vi "Alarma_EN50160_G02.vi"() -> ()   [LabVIEW 2018]
uses:
  Global/PQ_flags.vi
  Global/Alarmas_indicadores-LED.vi
  Global/estadoGeneradores.vi
  Global/Demo.vi
panel:
  in  "type specifier VI Refnum (for type only) 5":refnum<vi>
  in  "type specifier VI Refnum (for type only) 4":refnum<vi>
  in  "type specifier VI Refnum (for type only) 3":refnum<vi>
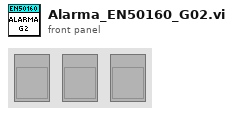
[diagram p1: front panel]
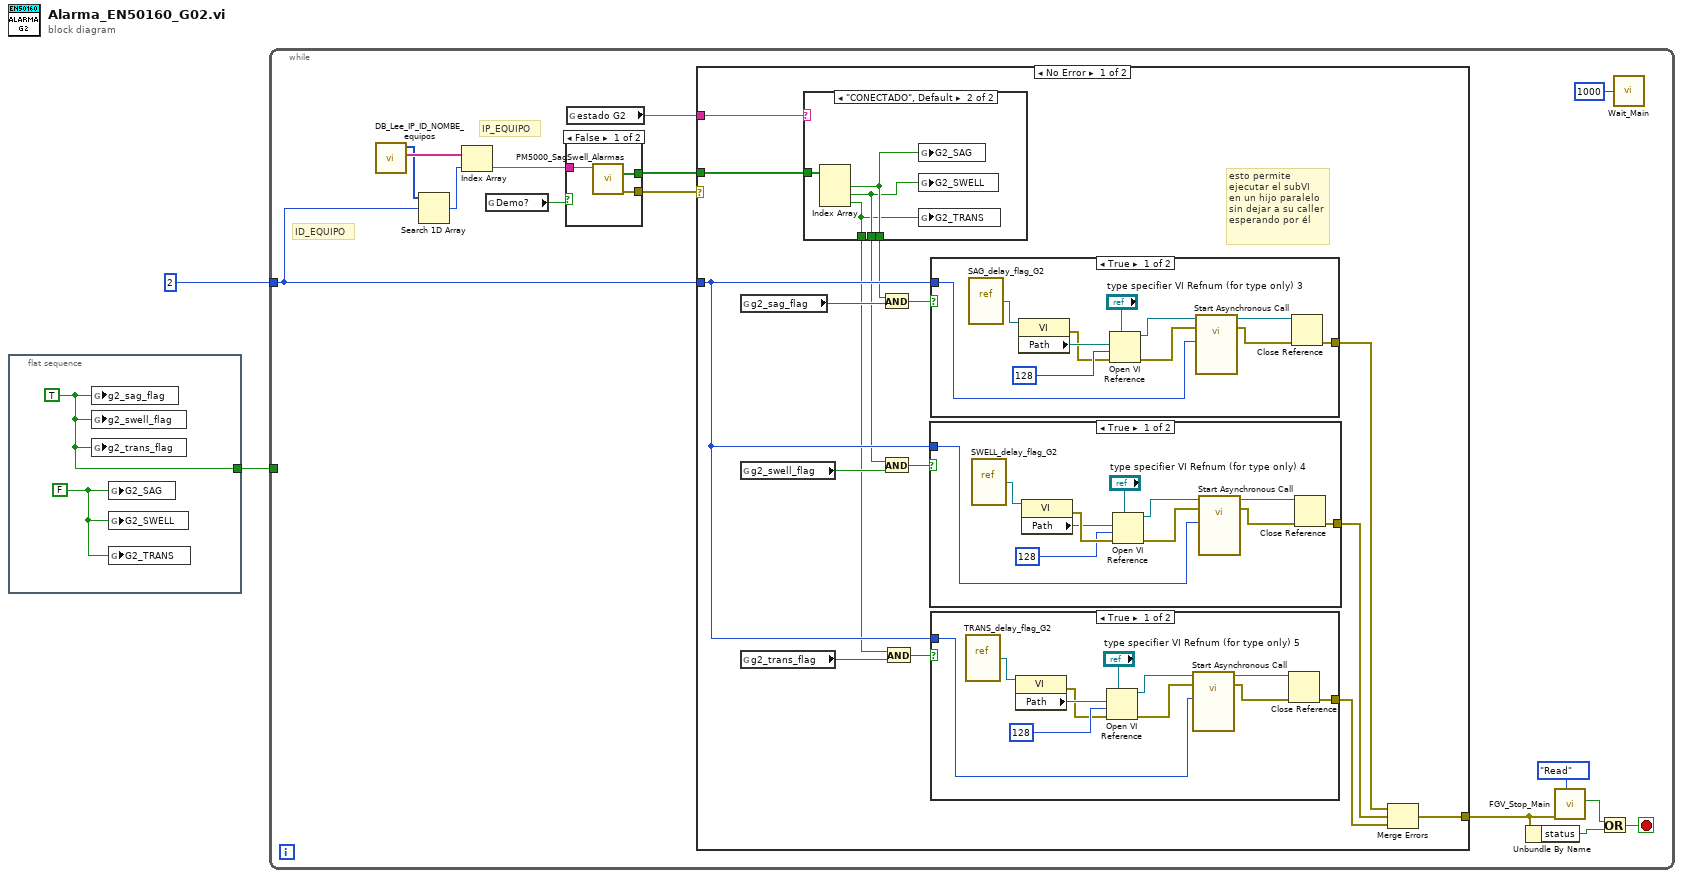
[diagram p0: block diagram]
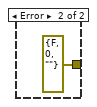
[diagram p6: hidden frame]
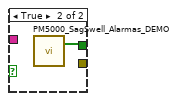
[diagram p7: hidden frame]
diagram:
  n1 = flat-sequence {
    tunnel: [w4] -> w2
    frame #0 {
      w3 = FALSE ("G1_SAG")
      w4 = TRUE ("sag_flag")
      n2 = global write "PQ_flags.vi" "g2_sag_flag"(w4) -> ()
      n3 = global write "PQ_flags.vi" "g2_swell_flag"(w4) -> ()
      n4 = global write "PQ_flags.vi" "g2_trans_flag"(w4) -> ()
      n5 = global write "Alarmas_indicadores-LED.vi" "G2_SAG"(w3) -> ()
      n6 = global write "Alarmas_indicadores-LED.vi" "G2_SWELL"(w3) -> ()
      n7 = global write "Alarmas_indicadores-LED.vi" "G2_TRANS"(w3) -> ()
    }
  }
  n8 = while {
    tunnel: w2 -> [_]
    tunnel: 2 ("element") -> [w6]
    stop <- w11 stop-if-true
    # "IP_EQUIPO"
    # "ID_EQUIPO"
    n9 = call "DB_Lee_IP_ID_NOMBE_equipos.vi"() -> ("IP_EQUIPO"=w18:string[], "ID_EQUIPO"=w16:i32[])  [unwired: 8 in, 2 out]
    n10 = Search 1D Array(1D array=w16, element=w6) -> (index of element=w17:i32)  [unwired: 1 in]
    n11 = Index Array(array=w18, index=w17) -> (element=w15:string)
    n12 = global read "Demo.vi" "Demo?"() -> (w5:bool)
    n13 = case shown="False" w5 {
      tunnel: [w76 w77] -> w19
      tunnel: w15 -> [w75 _]
      tunnel: [w74 _] -> w7
      frame False {
        n14 = call "PM5000_SagSwell_Alarmas.vi"("Network Path"=w75) -> ("error out"=w74:errorcluster, "PQ_Alarmas"=w76:bool[])  [unwired: 8 in, 1 out]
      }
      frame True {
        n15 = call "PM5000_SagSwell_Alarmas_DEMO.vi"() -> ("PQ_Alarmas 2"=w77:bool[])  [unwired: 14 in, 5 out]
      }
    }
    n16 = global read "estadoGeneradores.vi" "estado G2"() -> (w12:string)
    n17 = case shown="No Error" w7 {
      tunnel: w19 -> [w35 _]
      tunnel: w6 -> [w28 _]
      tunnel: w12 -> [w24 _]
      tunnel: [w20 errorcluster {"status"=FALSE, "code"=0, "source"=""} ("error IO")] -> w8
      frame No Error {
        # "esto permite \nejecutar el subVI\nen un hijo paralelo\nsin dejar a su caller\nesperando por él"
        n18 = global read "PQ_flags.vi" "g2_sag_flag"() -> (w31:bool)
        n19 = global read "PQ_flags.vi" "g2_swell_flag"() -> (w30:bool)
        n20 = global read "PQ_flags.vi" "g2_trans_flag"() -> (w29:bool)
        n21 = case shown="\"CONECTADO\", Default" w24 {
          tunnel: w35 -> [_ w39]
          tunnel: [_ w38] -> w27
          tunnel: [_ w37] -> w26
          tunnel: [_ w36] -> w25
          frame "DESCONECTADO" {
          }
          frame "CONECTADO", Default {
            n22 = Index Array(array=w39) -> (element #1=w38:bool, element #2=w37:bool, element #3=w36:bool)  [unwired: 3 in]
            n23 = global write "Alarmas_indicadores-LED.vi" "G2_SAG"(w38) -> ()
            n24 = global write "Alarmas_indicadores-LED.vi" "G2_SWELL"(w37) -> ()
            n25 = global write "Alarmas_indicadores-LED.vi" "G2_TRANS"(w36) -> ()
          }
        }
        n26 = And(x=w27, y=w31) -> (x .and. y?=w34:bool)
        n27 = And(x=w26, y=w30) -> (x .and. y?=w33:bool)
        n28 = And(x=w25, y=w29) -> (x .and. y?=w32:bool)
        n29 = case shown="True" w33 {
          tunnel: w28 -> [w52 _]
          tunnel: [w51 _] -> w22
          frame True {
            n30 = vi-ref "SWELL_delay_flag_G2.vi"() -> (w59:refnum<vi>)
            n31 = property class="VI"(reference=w59) -> (error out=w61:errorcluster, "Path"=w60:path)  [unwired: 1 in, 1 out]
            n32 = Open VI Reference(type specifier VI Refnum (for type only)="type specifier VI Refnum (for type only) 4", vi path=w60, options=128, error in (no error)=w61) -> (vi reference=w57:refnum<vi>, error out=w53:errorcluster)  [unwired: 2 in]
            n33 = call-by-ref "Start Asynchronous Call"(reference=w57, error in=w53, "ID_EQUIPO"=w52) -> (reference out=w54:refnum<vi>, error out=w55:errorcluster)  [unwired: 11 in]
            n34 = Close Reference(reference=w54, error in (no error)=w55) -> (error out=w51:errorcluster)
          }
          frame False {
          }
        }
        n35 = case shown="True" w34 {
          tunnel: w28 -> [w63 _]
          tunnel: [w62 _] -> w23
          frame True {
            n36 = vi-ref "SAG_delay_flag_G2.vi"() -> (w66:refnum<vi>)
            n37 = property class="VI"(reference=w66) -> (error out=w64:errorcluster, "Path"=w65:path)  [unwired: 1 in, 1 out]
            n38 = Open VI Reference(type specifier VI Refnum (for type only)="type specifier VI Refnum (for type only) 3", vi path=w65, options=128, error in (no error)=w64) -> (vi reference=w68:refnum<vi>, error out=w72:errorcluster)  [unwired: 2 in]
            n39 = call-by-ref "Start Asynchronous Call"(reference=w68, error in=w72, "ID_EQUIPO"=w63) -> (reference out=w71:refnum<vi>, error out=w70:errorcluster)  [unwired: 11 in]
            n40 = Close Reference(reference=w71, error in (no error)=w70) -> (error out=w62:errorcluster)
          }
          frame False {
          }
        }
        n41 = case shown="True" w32 {
          tunnel: w28 -> [w41 _]
          tunnel: [w40 _] -> w21
          frame True {
            n42 = vi-ref "TRANS_delay_flag_G2.vi"() -> (w44:refnum<vi>)
            n43 = property class="VI"(reference=w44) -> (error out=w42:errorcluster, "Path"=w43:path)  [unwired: 1 in, 1 out]
            n44 = Open VI Reference(type specifier VI Refnum (for type only)="type specifier VI Refnum (for type only) 5", vi path=w43, options=128, error in (no error)=w42) -> (vi reference=w46:refnum<vi>, error out=w50:errorcluster)  [unwired: 2 in]
            n45 = call-by-ref "Start Asynchronous Call"(reference=w46, error in=w50, "ID_EQUIPO"=w41) -> (reference out=w49:refnum<vi>, error out=w48:errorcluster)  [unwired: 11 in]
            n46 = Close Reference(reference=w49, error in (no error)=w48) -> (error out=w40:errorcluster)
          }
          frame False {
          }
        }
        n47 = Merge Errors(w23, w22, w21) -> (w20:errorcluster)
      }
      frame Error {
      }
    }
    n48 = Unbundle By Name(w8) -> ("status"=w9:bool)
    n49 = call "FGV_Stop_Main.vi"("Action"=enum16{"Read", "Write"}."Read", "Error In (no error)"=w8) -> ("Var Out"=w10:bool)  [unwired: 8 in, 1 out]
    n50 = Or(x=w10, y=w9) -> (x .or. y?=w11:bool)
    n51 = call "Wait_Main.vi"("Wait time (msec)"=u32 1000) -> ()  [unwired: 5 in]
  }
